vi "Clamp.vi"(6 "Axis":T1, 8 "error in (no error)":errorcluster, 11 "Instrument.VRM in":refnum<class "Instrument.OxfordVRM.lvclass">) -> (0 "error out":errorcluster, 2 "Response":string, 3 "Instrument.VRM out":refnum<class "Instrument.OxfordVRM.lvclass">)   [LabVIEW 2016, in "Instrument.OxfordVRM.lvclass"]
uses:
  Instrument.OxfordVRM.lvclass
  Typedefs/VRM Magnet Axis--Enum.ctl
  Typedefs/Instrument.VRM.Commands-enum.ctl
  <instrlib>/Mercury iXX/Public/Libraries/Magnet/Controls/PSU Actions.ctl
  Typedefs/VRM Action-Axis--Cluster.ctl
  <instrlib>/Mercury iXX/Public/Libraries/Magnet.lvlib
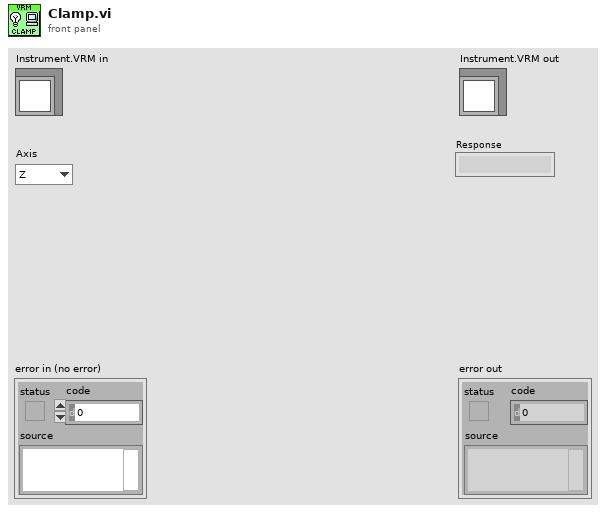
[diagram p1: front panel]
types:
  T1 = typedef "Instrument.OxfordVRM.lvclass/VRM Magnet Axis--Enum.ctl" = enum16{"Z", "X", "Y", "ALL"}
  T2 = typedef "Instrument.OxfordVRM.lvclass/VRM Action-Axis--Cluster.ctl" = cluster{"PSU Act Stat":T3, "Axis":T1}
  T3 = typedef "Mercury iXX.lvlib/Magnet.lvlib/PSU Actions.ctl" = string
  T4 = typedef "Instrument.OxfordVRM.lvclass/Instrument.VRM.Commands-enum.ctl" = enum16{"setAction", "setTarget", "setMagnetField", "getStatus", "getTarget", "getMagnetField"}
  T5 = cluster{"Holding":bool, "Ramp to Setpoint":bool, "Ramp to Zero":bool, "Clamp":bool}
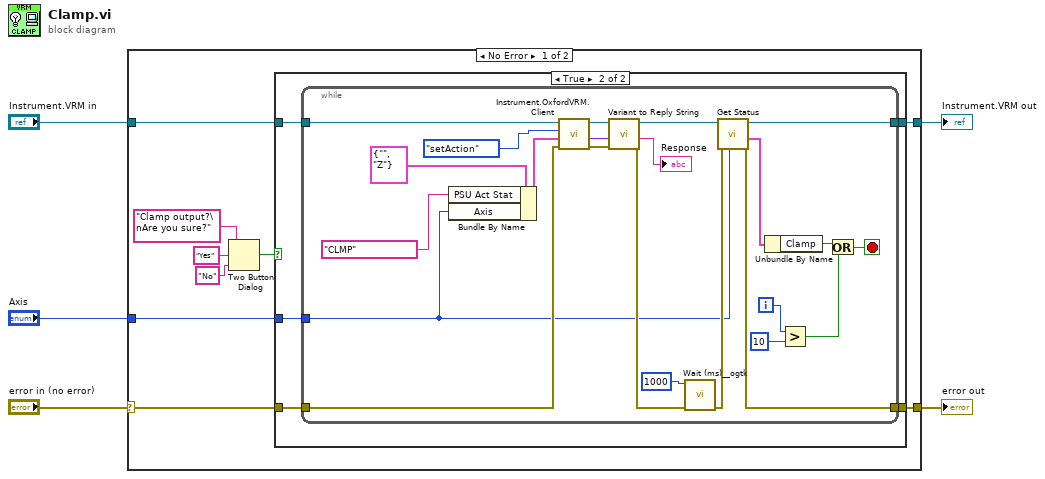
[diagram p0: block diagram]
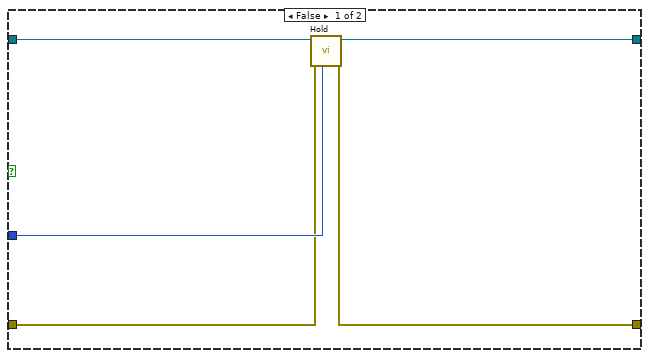
[diagram p2: hidden frame]
diagram:
  n1 = case shown="No Error" "error in (no error)" {
    selector: "error in (no error)" -> [w13 w49]
    tunnel: [w11 w49] -> w4
    tunnel: [w12 w48] -> w2
    tunnel: "Instrument.VRM in" -> [w14 w48]
    tunnel: "Axis" -> [w10 _]
    frame No Error {
      n2 = Two Button Dialog(message="Clamp output?\nAre you sure?", 1:"No" ("F button name (\"Cancel\")"), 2:"Yes" ("T button name (\"OK\")")) -> (T button?=w6:bool)
      n3 = case shown="True" w6 {
        tunnel: w14 -> [w18 w24]
        tunnel: w13 -> [w15 w23]
        tunnel: [w17 w22] -> w12
        tunnel: [w16 w21] -> w11
        tunnel: w10 -> [w19 w20]
        frame False {
          n4 = call "Hold.vi"("Axis"=w19, "error in (no error)"=w15, "Instrument.VRM in"=w18) -> ("error out"=w16:errorcluster, "Instrument.VRM out"=w17:refnum<class "Instrument.OxfordVRM.lvclass">)  [unwired: 6 in, 1 out]
        }
        frame True {
          n5 = while {
            tunnel: w24 -> [w43]
            tunnel: [w45] -> w22
            tunnel: w23 -> [w47]
            tunnel: [w26] -> w21
            tunnel: w20 -> [w25]
            i -> [w38]
            stop <- w39 stop-if-true
            n6 = Bundle By Name(cluster=T2 {"PSU Act Stat"="", "Axis"=enum."Z"}, "PSU Act Stat"=T3 "CLMP", "Axis"=w25) -> (w29:T2)
            n7 = call "Instrument.OxfordVRM.Client.vi"("error in (no error)"=w47, "Data"=w29, "Commands"=Instrument.VRM.Commands-enum."setAction", "Instrument.VRM in"=w43) -> ("error out"=w35:errorcluster, "Data out"=w34:variant, "Instrument.VRM out"=w37:refnum<class "Instrument.OxfordVRM.lvclass">)  [unwired: 5 in]
            n8 = call "Variant to Reply String.vi"("error in (no error)"=w35, "Data"=w34, "Instrument.VRM in"=w37) -> ("error out"=w33:errorcluster, "Reply"=→"Response":string, "Instrument.VRM out"=w36:refnum<class "Instrument.OxfordVRM.lvclass">)  [unwired: 6 in]
            n9 = call <userlib>:"Wait (ms)__ogtk.vi"("error in (no error)"=w33, "milliseconds to wait"=u32 1000) -> ("error out"=w44:errorcluster)  [unwired: 8 in, 1 out]
            n10 = call "Get Status.vi"("Axis"=w25, "error in (no error)"=w44, "Instrument.VRM in"=w36) -> ("error out"=w26:errorcluster, "Status (ALL)"=w46:T5, "Instrument.VRM out"=w45:refnum<class "Instrument.OxfordVRM.lvclass">)  [unwired: 5 in, 1 out]
            n11 = Unbundle By Name(w46) -> ("Clamp"=w40:bool)
            n12 = Greater?(x=w38, y=10) -> (0:w41:bool)
            n13 = Or(x=w40, y=w41) -> (x .or. y?=w39:bool)
          }
        }
      }
    }
    frame Error {
    }
  }
  "error out" <- w4
  "Instrument.VRM out" <- w2
